vi "recurse.vi"(11 "reference":refnum<vi>) -> (3 "concatenated string":string)   [LabVIEW 2024]
panel:
  out "error out":errorcluster
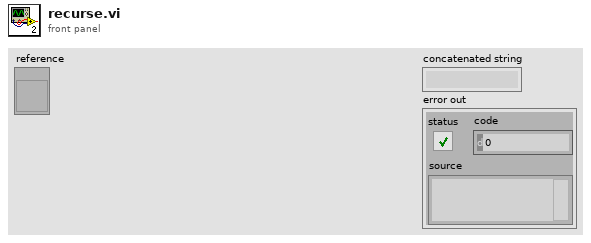
[diagram p1: front panel]
types:
  T1 = enum32{"not a typedef", "typedef", "strict typedef", "class private data"}
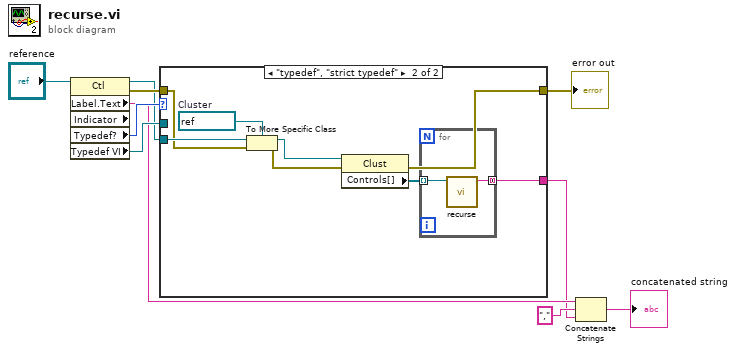
[diagram p0: block diagram]
diagram:
  n1 = property class="Ctl" props=["Label", "Text", "Indicator", "Typedef?", "Typedef VI"](reference="reference") -> (reference out=w5:refnum<vi>, error out=w6:errorcluster, "Label.Text"=w7:string, "Typedef?"=w10:T1, "Typedef VI"=w9:refnum<vi>)  [unwired: 1 in, 1 out]
  n2 = case shown="\"typedef\", \"strict typedef\"" w10 {
    tunnel: w9 -> [_ _]
    tunnel: w6 -> [w11 w14]
    tunnel: [w11 w12] -> w1
    tunnel: w5 -> [_ w18]
    tunnel: [_ w17] -> w2
    frame "not a typedef", Default {
    }
    frame "typedef", "strict typedef" {
      w19 = refnum<vi> refnum  # Cluster
      n3 = To More Specific Class(target class=w19, reference=w18, error in=w14) -> (specific class reference=w16:refnum<vi>, error out=w13:errorcluster)
      n4 = property class="Clust"(reference=w16, error in=w13) -> (error out=w12:errorcluster, "Controls[]"=w15:refnum<vi>[])  [unwired: 1 out]
      n5 = for {
        tunnel: w15 -> [w21] mode=indexing
        tunnel: [w20] -> w17 mode=concatenating
        n6 = call "recurse.vi"("reference"=w21) -> ("concatenated string"=w20:string)  [unwired: 10 in]
      }
    }
  }
  "error out" <- w1
  n7 = Concatenate Strings(w7, ",", w2) -> (→"concatenated string":string)
